vi "addOutputChannels.vi"(8 "error in":errorcluster, 10 "WaveformTask ID":T1 format="%.0x", 11 "CustomDevice Ref":T1 format="%.0x") -> (0 "error out":errorcluster, 2 "Array":bool[](array[boolean]), 3 "'Analog Input' Section Refs":refnum<k24>[](array[refnum]))   [LabVIEW 2014, in "Waveform-Processing-Custom-Device System Explorer.lvlib"]
uses:
  Waveform-Processing-Custom-Device System Explorer.lvlib
  <vilib>/NI Veristand/Custom Device API/Custom Device Item Ref.ctl
  NationalInstruments.VeriStand.SystemStorage
  <vilib>/NI Veristand/Custom Device Tools/Custom Device Utility Library/Custom Device Utility Library.lvlib
  <vilib>/NI Veristand/Custom Device API/Custom Device API.lvlib
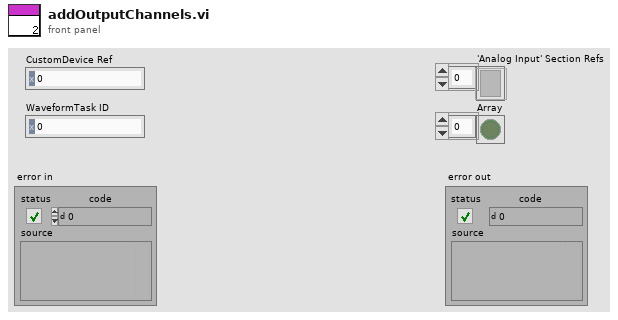
[diagram p1: front panel]
types:
  T1 = typedef "Custom Device API.lvlib/Custom Device Item Ref.ctl" = u64
  T2 = typedef "Custom Device API.lvlib/Custom Device Pointer.ctl" = refnum<k24>
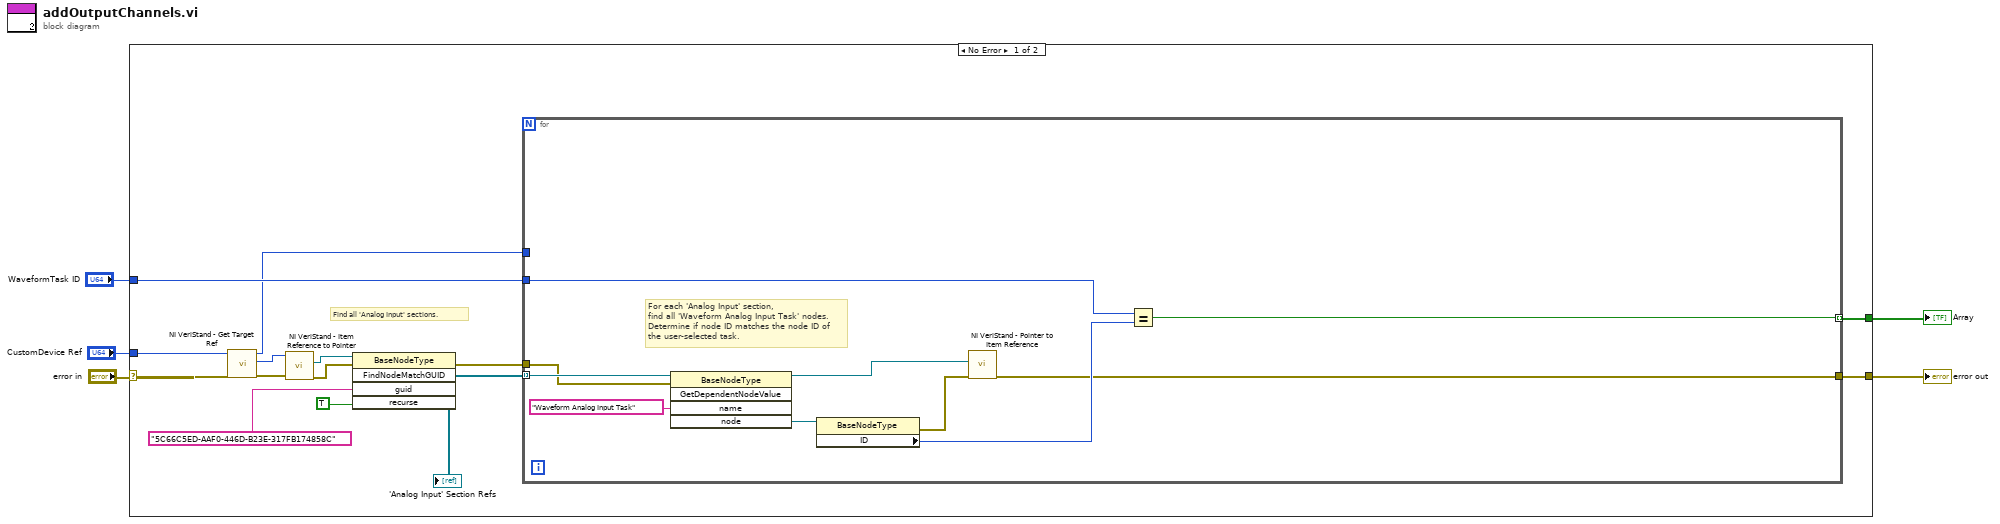
[diagram p0: block diagram]
diagram:
  n1 = case shown="No Error" "error in" {
    selector: "error in" -> [w19 w30]
    tunnel: [w7 w30] -> w4
    tunnel: "CustomDevice Ref" -> [w18 _]
    tunnel: "WaveformTask ID" -> [w17 _]
    tunnel: [w6 _] -> w1
    frame No Error {
      # "Find all 'Analog Input' sections."
      n2 = call <vilib>:"NI VeriStand - Get Target Ref.vi"("error in"=w19, "Item Ref in"=w18) -> ("error out"=w15:errorcluster, "Target Ref"=w14:T1, "Item Ref out"=w16:T1)  [unwired: 6 in, 1 out]
      n3 = call <vilib>:"NI VeriStand - Item Reference to Pointer.vi"("error in (no error)"=w15, "Item Ref in"=w14) -> ("error out"=w12:errorcluster, "Node Pointer"=w13:T2)  [unwired: 6 in, 2 out]
      n4 = invoke class="BaseNodeType" method="FindNodeMatchGUID"(reference=w13, error in=w12, "guid"="5C66C5ED-AAF0-446D-B23E-317FB174858C" ("Item GUID"), "recurse"=TRUE ("Find All? (T)")) -> (error out=w8:errorcluster, "FindNodeMatchGUID"=w9:refnum<k24>[])  [unwired: 1 in, 3 out]
      "'Analog Input' Section Refs" <- w9
      n5 = for {
        tunnel: w17 -> [w29]
        tunnel: w16 -> [_]
        tunnel: w9 -> [w28] mode=indexing
        tunnel: w8 -> [w27]
        tunnel: [w21] -> w7
        tunnel: [w20] -> w6 mode=indexing
        # "For each 'Analog Input' section, \nfind all 'Waveform Analog Input Task' nodes.\nDetermine if node ID matches the node ID of \nthe user-selected task."
        n6 = invoke class="BaseNodeType" method="GetDependentNodeValue"(reference=w28, error in=w27, "name"="Waveform Analog Input Task" ("Property Name")) -> (reference out=w23:refnum<k24>, "node"=w25:refnum<k24>)  [unwired: 2 in, 3 out]
        n7 = property class="BaseNodeType"(reference=w25) -> (error out=w22:errorcluster, "ID"=w24:u64)  [unwired: 1 in, 1 out]
        n8 = call <vilib>:"NI VeriStand - Pointer to Item Reference.vi"("error in (no error)"=w22, "Node Pointer"=w23) -> ("error out"=w21:errorcluster)  [unwired: 8 in, 1 out]
        n9 = Equal?(x=w29, y=w24) -> (x = y?=w20:bool)
      }
    }
    frame Error {
    }
  }
  "error out" <- w4
  "Array" <- w1
